vi "TDMSAddBlankElem1d.vi"(1 "input string array":string[](array[string])) -> (0 "output string array with blank element at the beginning":string[](array[string]))   [LabVIEW 2020]
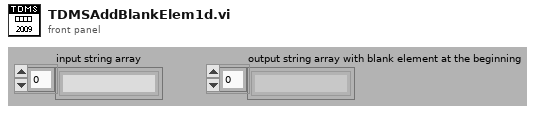
[diagram p1: front panel]
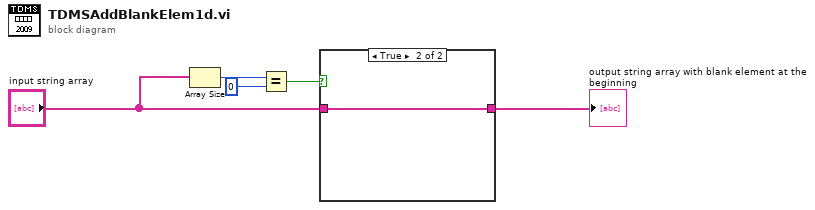
[diagram p0: block diagram]
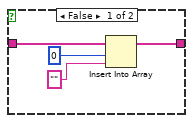
[diagram p2: hidden frame]
diagram:
  n1 = Array Size(array="input string array") -> (size(s)=w5:i32)
  n2 = Equal?(x=w5, y=0) -> (x = y?=w3:bool)
  n3 = case shown="True" w3 {
    tunnel: "input string array" -> [w7 w10]
    tunnel: [w6 w10] -> w1
    frame False {
      n4 = Insert Into Array(array=w7, index=0, new element="" ("new element/subarray")) -> (w6:string[])
    }
    frame True {
    }
  }
  "output string array with blank element at the beginning" <- w1
